vi "Convert Mouse Button Event Data.vi"(11 "Event Data":u8[](array[numeric])) -> (3 "Mouse Button Event":T1)   [LabVIEW 2014, in "LibSDL2.lvlib"]
uses:
  LibSDL2.lvlib
  Controls/Mouse Button Event.ctl
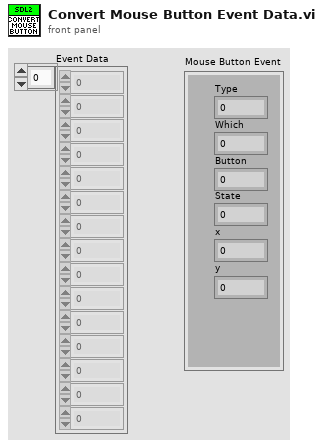
[diagram p1: front panel]
types:
  T1 = typedef "LibSDL2.lvlib/Mouse Button Event.ctl" = cluster{"Type":u8, "Which":u8, "Button":u8, "State":u8, "x":u16, "y":u16}
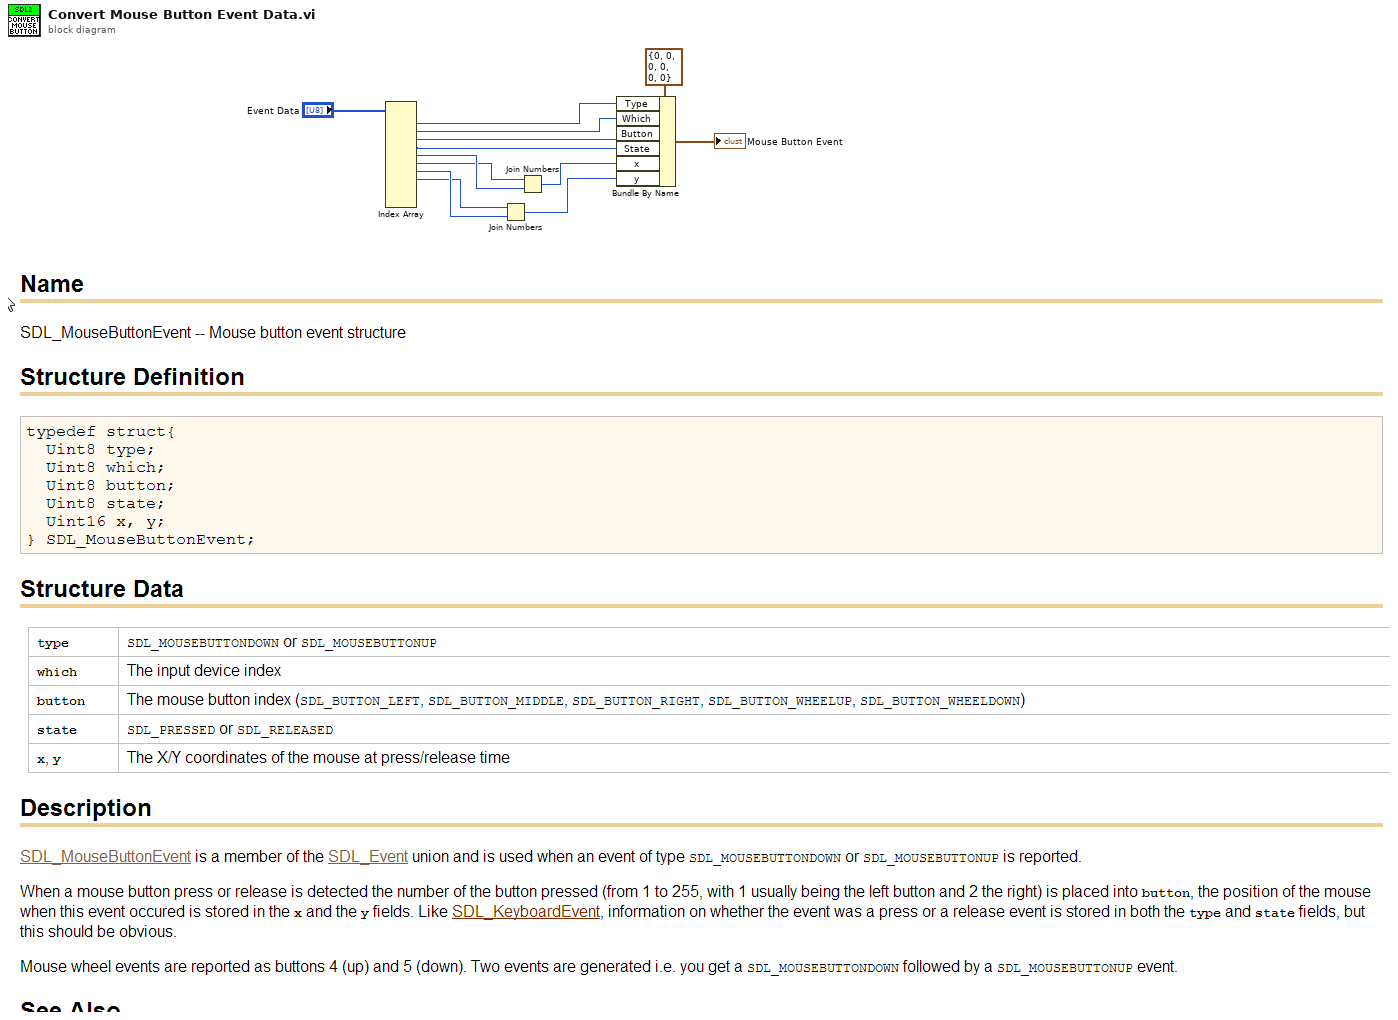
[diagram p0: block diagram]
diagram:
  n1 = Index Array(array="Event Data") -> (element #1=w10:u8, element #2=w11:u8, element #3=w12:u8, element #4=w7:u8, element #5=w6:u8, element #6=w5:u8, element #7=w3:u8, element #8=w2:u8)  [unwired: 11 in, 3 out]
  n2 = Join Numbers(hi=w2, lo=w3) -> ((hi.lo)=w1:u16)
  n3 = Join Numbers(hi=w5, lo=w6) -> ((hi.lo)=w4:u16)
  n4 = Bundle By Name(cluster=T1 {"Type"=0, "Which"=0, "Button"=0, "State"=0, "x"=0, "y"=0} ("Mouse Button Event"), "Type"=w10, "Which"=w11, "Button"=w12, "State"=w7, "x"=w4, "y"=w1) -> (→"Mouse Button Event":T1)
